vi "Existing_System.vi"() -> ()   [LabVIEW 2023]
uses:
  <vilib>/NI/Modbus Library/API/Wrapper/Create TCP Slave.vi
  <vilib>/NI/Modbus Library/API/Slave/Modbus Slave.lvclass
  <vilib>/NI/Modbus Library/API/Wrapper/API Main.lvlib
panel:
  out "Operation":bool
  out "Stop":bool
  out "Actuations":dbl
  out "Change Plunger":bool
  in  "Run":bool
  out "Passes":dbl
  out "Fails":dbl
  out "Total":dbl
  out "?":dbl
  out "Status":bool
  # "Cap Sealer Indicators"
  # "Modbus Slave"
  # "Change Plunger Indicator"
  # "Bottle Cap  Sealer Machine Operations"
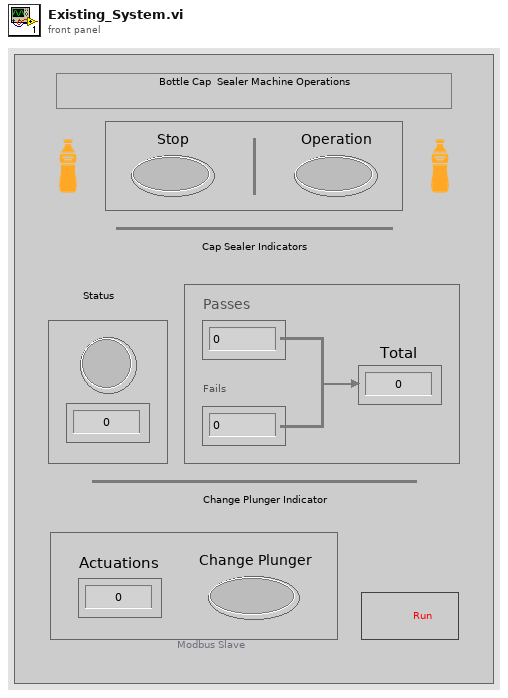
[diagram p1: front panel]
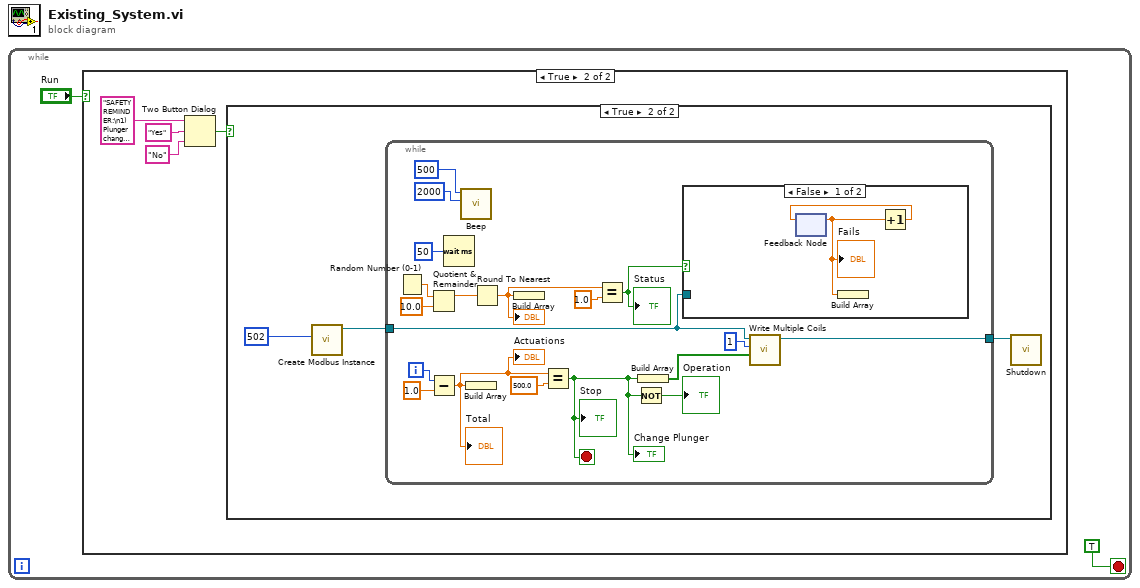
[diagram p0: block diagram]
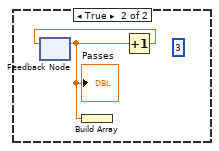
[diagram p4: hidden frame]
diagram:
  n1 = while {
    stop <- TRUE stop-if-true
    n2 = case shown="True" "Run" {
      frame False {
      }
      frame True {
        n3 = Two Button Dialog(message="SAFETY REMINDER:\n1) Plunger changed?\n2) Is it safe to proceed?", 1:"No" ("button name (\"OK\")"), 2:"Yes" ("T button name (\"OK\")")) -> (T button?=w3:bool)
        n4 = case shown="True" w3 {
          frame False {
          }
          frame True {
            n5 = call-poly <vilib>:"Create Modbus Instance.vi"("port (502)"=u16 502) -> ("TCP slave instance"=w8:refnum<class "Modbus Slave.lvclass">)  [unwired: 9 in, 1 out]
            n6 = while {
              tunnel: w8 -> [w14]
              tunnel: [w15] -> w7
              i -> [w18]
              stop <- w11 stop-if-true
              n7 = Random Number (0-1)() -> (number: 0 to 1=w28:dbl)
              n8 = Quotient & Remainder(x=w28, y=10.0) -> (x-y*floor(x/y)=w26:dbl)  [unwired: 1 out]
              n9 = Subtract(x=w18, y=1.0) -> (x-y=w12:dbl)
              "Total" <- w12
              "Actuations" <- w12
              n10 = Wait (ms)(milliseconds to wait=u32 50) -> ()  [unwired: 1 out]
              n11 = call <vilib>:"Beep.vi"("duration (msec)"=u32 2000, "frequency (Hz)"=u32 500) -> ()  [unwired: 10 in]
              n12 = Build Array(w12) -> ()  [unwired: 1 out]
              n13 = Round To Nearest(number=w26) -> (nearest integer value=w13:dbl)
              "?" <- w13
              n14 = Build Array(w13) -> ()  [unwired: 1 out]
              n15 = Equal?(x=w12, y=500.0) -> (x = y?=w11:bool)
              "Change Plunger" <- w11
              "Stop" <- w11
              n16 = Equal?(x=w13, y=1.0) -> (x = y?=w20:bool)
              "Status" <- w20
              n17 = Not(x=w11) -> (.not. x?=→"Operation":bool)
              n18 = Build Array(w11) -> (w10:bool[])
              n19 = case shown="False" w20 {
                tunnel: w14 -> [_ _]
                frame False {
                  n20 = feedback #1() -> (w29:dbl)  [unwired: 1 in]
                  "Fails" <- w29
                  n21 = Build Array(w29) -> ()  [unwired: 1 out]
                  n22 = Increment(x=w29) -> (x+1=w30:dbl)
                  n23 = feedback-in #1(w30) -> ()
                }
                frame True {
                  (unwired) u16 3 ("address")
                  n24 = feedback #2() -> (w31:dbl)  [unwired: 1 in]
                  "Passes" <- w31
                  n25 = Build Array(w31) -> ()  [unwired: 1 out]
                  n26 = Increment(x=w31) -> (x+1=w32:dbl)
                  n27 = feedback-in #2(w32) -> ()
                }
              }
              n28 = call-dynamic "Write Multiple Coils.vi"("coils to write"=w10, "starting address"=u16 1 ("address"), "Modbus slave in"=w14) -> ("Modbus slave out"=w15:refnum<class "Modbus Slave.lvclass">)  [unwired: 7 in, 1 out]
            }
            n29 = call-dynamic "Shutdown.vi"("Modbus slave in"=w7) -> ()  [unwired: 10 in, 1 out]
          }
        }
      }
    }
  }
